vi "FTW-Connector-Close.vi"(0 "FTW Actor Connector":refnum<class "FTW-ActorConnector.lvclass">, 11 "error in":errorcluster) -> (15 "error out":errorcluster)   [LabVIEW 2015, in "FTW-ActorConnector.lvclass"]
uses:
  FTW-ActorConnector.lvclass
  FTW-ActorConnector.lvclass/FTW-ActorConnector.ctl
  Request/FTW-Request.lvclass
panel:
  # "Inputs"
  # "Outputs"
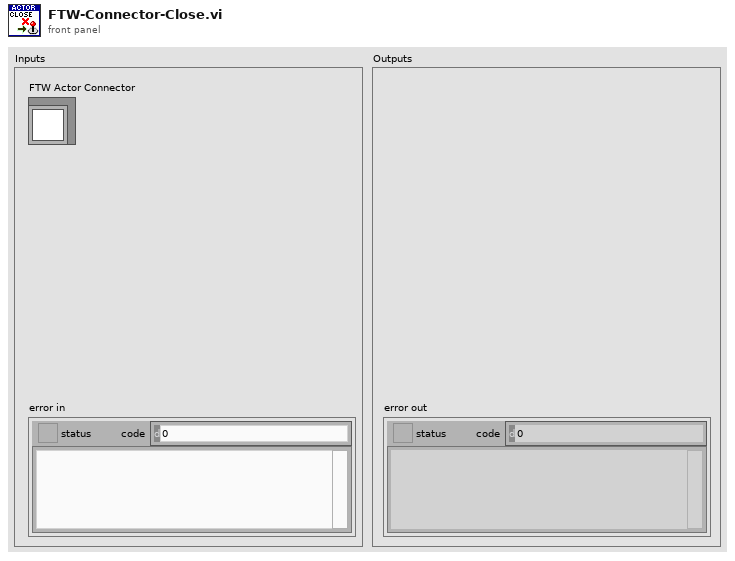
[diagram p1: front panel]
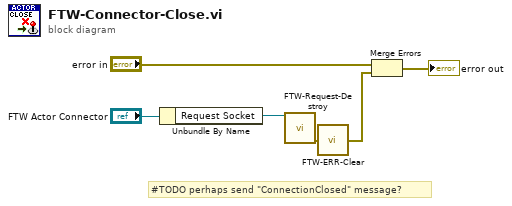
[diagram p0: block diagram]
diagram:
  # "#TODO perhaps send \"ConnectionClosed\" message?"
  n1 = Unbundle By Name("FTW Actor Connector") -> ("Request Socket"=w3:refnum<class "FTW-Request.lvclass">)
  n2 = call "FTW-Request-Destroy.vi"("FTW-Request In"=w3) -> ("error out"=w2:errorcluster)  [unwired: 14 in]
  n3 = call "FTW-ERR-Clear.vi"("error to snuff"=w2) -> ("no error"=w1:errorcluster)
  n4 = Merge Errors("error in", w1) -> (→"error out":errorcluster)
